vi "close_all_channels_except.vi"(9 "Channel":enum16{"1", "2", "3", "4", "5", "6", "7", "8"}[](array[ring]), 10 "Flowboard":enum16{"A", "B", "C"}[](array[ring]), 11 "Channels to Exclude":u16[](array[ring]) items=["A1", "A2", "A3", "A4", "A5", "A6", "A7", "A8", "B1", "B2", "B3", "B4", "B5", "B6", "B7", "B8", "C1", "C2", "C3", "C4", "C5", "C6", "C7", "C8"]) -> ()   [LabVIEW 2016]
panel:
  out "Channel Name":u16(ring) items=["A1", "A2", "A3", "A4", "A5", "A6", "A7", "A8", "B1", "B2", "B3", "B4", "B5", "B6", "B7", "B8", "C1", "C2", "C3", "C4", "C5", "C6", "C7", "C8"]
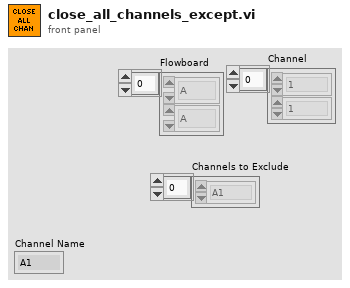
[diagram p1: front panel]
types:
  T1 = enum16{"Release", "Create", "Send", "Wait", "Cancel"}
  T2 = cluster{enum16{"A", "B", "C"}[], enum16{"1", "2", "3", "4", "5", "6", "7", "8"}[], bool[]}
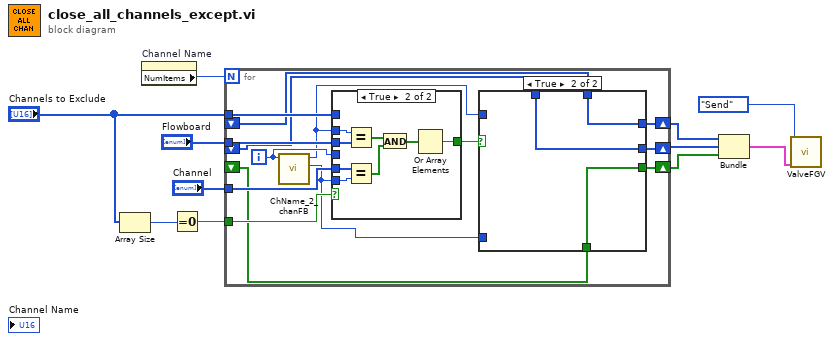
[diagram p0: block diagram]
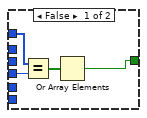
[diagram p2: hidden frame]
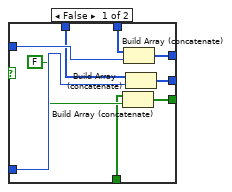
[diagram p3: hidden frame]
diagram:
  n1 = Array Size(array="Channels to Exclude") -> (size(s)=w9:i32)
  n2 = property on="Channel Name" class="Ring (strict)"() -> ("NumItems"=w11:u32)  [unwired: 2 in, 2 out]
  n3 = Equal To 0?(x=w9) -> (x = 0?=w8:bool)
  n4 = for {
    N: w11 -> [_]
    tunnel: "Channels to Exclude" -> [w21]
    tunnel: w8 -> [w23]
    tunnel: "Flowboard" -> [w25]
    tunnel: "Channel" -> [w24]
    shift-right: [w17] -> w4
    shift-left: _ -> [w13]
    shift-right: [w16] -> w5
    shift-left: _ -> [w14]
    shift-right: [w15] -> w3
    shift-left: _ -> [w12]
    i -> [w20]
    n5 = call "ChName_2_chanFB.vi"("Channel Name"=w20) -> ("Channel Out"=w18:enum16{"1", "2", "3", "4", "5", "6", "7", "8"}, "Flowboard Out"=w19:enum16{"A", "B", "C"})  [unwired: 9 in]
    n6 = case shown="True" w23 {
      tunnel: w19 -> [_ w30]
      tunnel: w25 -> [_ w37]
      tunnel: w24 -> [_ w36]
      tunnel: w18 -> [_ w35]
      tunnel: [w26 w31] -> w22
      tunnel: w21 -> [w29 _]
      tunnel: w20 -> [w28 _]
      frame False {
        n7 = Equal?(x=w29, y=w28) -> (x = y?=w27:bool[])
        n8 = Or Array Elements(Boolean array=w27) -> (logical OR=w26:bool)
      }
      frame True {
        n9 = Equal?(x=w30, y=w37) -> (x = y?=w34:bool[])
        n10 = Equal?(x=w36, y=w35) -> (x = y?=w33:bool[])
        n11 = And(x=w34, y=w33) -> (x .and. y?=w32:bool[])
        n12 = Or Array Elements(Boolean array=w32) -> (logical OR=w31:bool)
      }
    }
    n13 = case shown="True" w22 {
      tunnel: w19 -> [w44 _]
      tunnel: w18 -> [w46 _]
      tunnel: [w45 w48] -> w17
      tunnel: [w43 w49] -> w16
      tunnel: [w41 w47] -> w15
      tunnel: w14 -> [w40 w49]
      tunnel: w13 -> [w39 w48]
      tunnel: w12 -> [w38 w47]
      frame False {
        n14 = Build Array (concatenate)(w38, FALSE ("State")) -> (w41:bool[])
        n15 = Build Array (concatenate)(w40, w44) -> (w43:enum16{"A", "B", "C"}[])
        n16 = Build Array (concatenate)(w39, w46) -> (w45:enum16{"1", "2", "3", "4", "5", "6", "7", "8"}[])
      }
      frame True {
      }
    }
  }
  n17 = Bundle(w5, w4, w3) -> (w1:T2)  [unwired: 1 in]
  n18 = call "ValveFGV.vi"("Valve Data"=w1, "Action"=T1."Send") -> ()  [unwired: 6 in, 4 out]
